vi "VI Execution Properties.vi"() -> ()   [LabVIEW 2023]
doc: "SubVI Inlining eliminates subVI calling overhead and enables additional optimizations, while maintaining source-code modularity. This example compares the run-time performance of an inline subVI against a normal subVI with debugging, a normal subVI without debugging, a subroutine subVI, and the primitive itself."
panel:
  out "Debugging Disabled":dbl
  out "Inlined":dbl
  out "Subroutine Priority":dbl
  out "Debugging Enabled":dbl
  out "Direct Function Call":dbl
  out "Data":dbl[](array[numeric])
  # "Overview: Demonstrates the performance effects of various VI Properties > Execution settings.\nInstructions:\n1. Close all open VIs except this one.\n2. Run the VI. It may take several seconds to complete. See the block diagram for more information on these benchmark values."
  # "Execution Times (ns)"
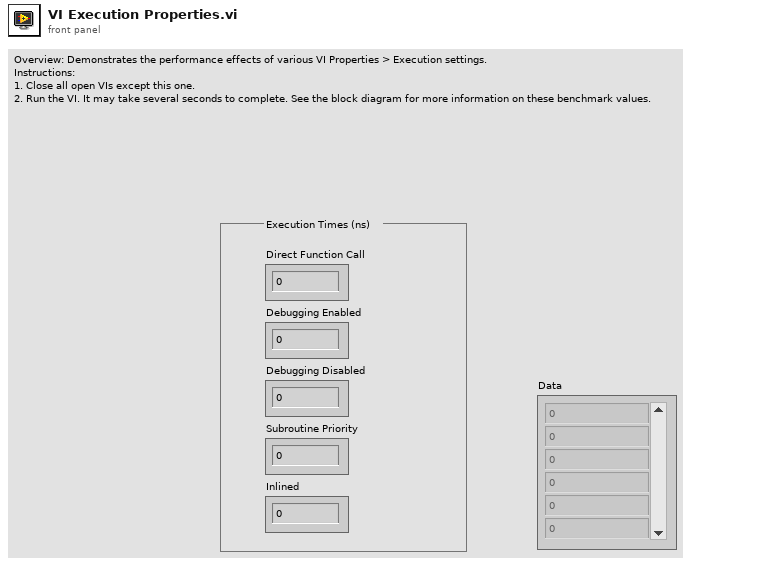
[diagram p1: front panel]
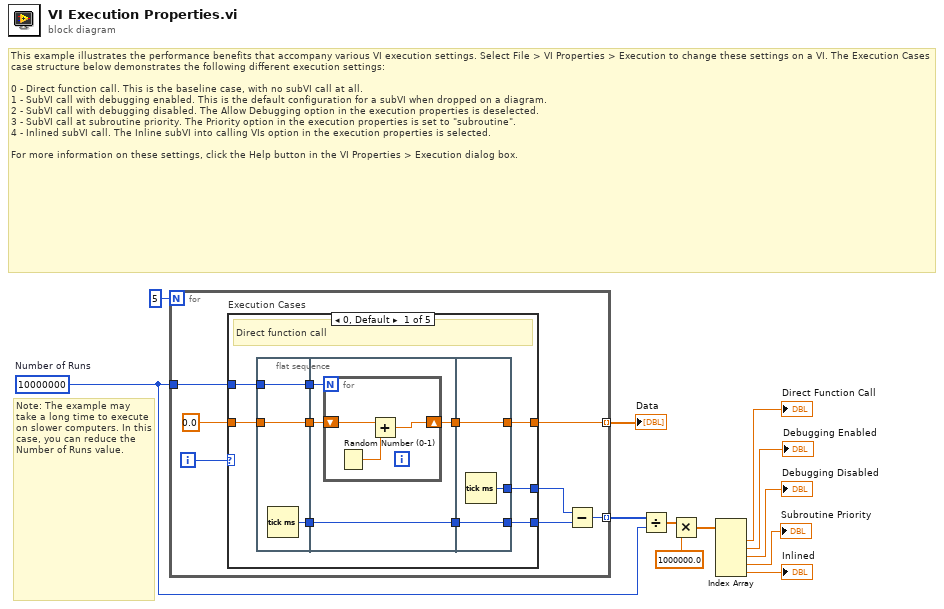
[diagram p0: block diagram]
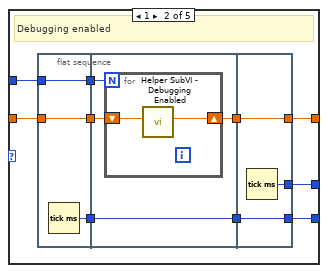
[diagram p2: hidden frame]
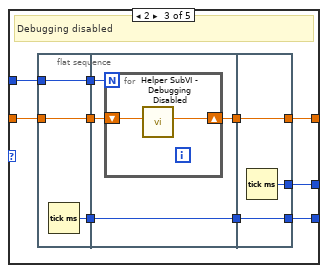
[diagram p3: hidden frame]
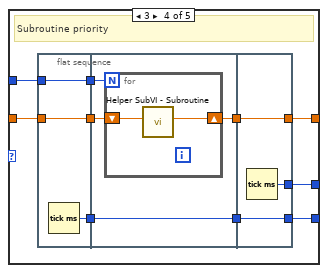
[diagram p4: hidden frame]
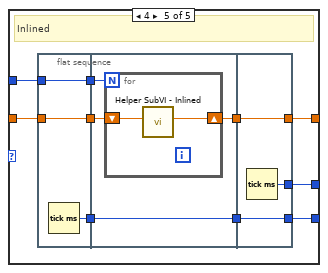
[diagram p5: hidden frame]
diagram:
  w10 = 10000000  # Number of Runs
  # "Note: The example may take a long time to execute on slower computers. In this case, you can reduce the Number of Runs value."
  # "This example illustrates the performance benefits that accompany various VI execution settings. Select File > VI Properties > Execution to change these settings on a VI. The Execution Cases case structure below demonstrates the following different execution settings:\n\n0 - Direct function call. This is the baseline case, with no subVI call at all.\n1 - SubVI call with debugging enabled. This is the default configuration for a subVI when dropped on a diagram.\n2 - SubVI call with debugging disabled. The Allow Debugging option in the execution properties is deselected.\n3 - SubVI call at subroutine priority. The Priority option in the execution properties is set to \"subroutine\".\n4 - Inlined subVI call. The Inline subVI into calling VIs option in the execution properties is selected.\n\nFor more information on these settings, click the Help button in the VI Properties > Execution dialog box."
  n1 = for {
    N: 5 -> [_]
    tunnel: [w17] -> w11 mode=indexing
    tunnel: w10 -> [w15]
    tunnel: [w16] -> w12 mode=indexing
    i -> [w13]
    n2 = case "Execution Cases" shown="0, Default" w13 {
      tunnel: [w24 w47 w69 w91 w113] -> w19
      tunnel: [w23 w46 w68 w90 w112] -> w18
      tunnel: [w22 w45 w67 w89 w111] -> w16
      tunnel: w15 -> [w21 w44 w66 w88 w110]
      tunnel: 0.0 -> [w20 w43 w65 w87 w109]
      frame 0, Default {
        # "Direct function call"
        n3 = flat-sequence {
          tunnel: [w32] -> w29
          tunnel: [w31] -> w28
          tunnel: w21 -> [w31]
          tunnel: [w30] -> w27
          tunnel: w20 -> [w30]
          tunnel: [w36] -> w26
          tunnel: w29 -> [w36]
          tunnel: w28 -> [w35]
          tunnel: w27 -> [w34]
          tunnel: [w33] -> w25
          tunnel: w26 -> [w42]
          tunnel: [w42] -> w23
          tunnel: [w41] -> w24
          tunnel: [w40] -> w22
          tunnel: w25 -> [w40]
          frame #0 {
            n4 = Tick Count (ms)() -> (millisecond timer value=w32:u32)
          }
          frame #1 {
            n5 = for {
              N: w35 -> [_]
              shift-right: [w38] -> w33
              shift-left: w34 -> [w39]
              n6 = Random Number (0-1)() -> (number: 0 to 1=w37:dbl)
              n7 = Add(x=w39, y=w37) -> (x+y=w38:dbl)
            }
          }
          frame #2 {
            n8 = Tick Count (ms)() -> (millisecond timer value=w41:u32)
          }
        }
      }
      frame 1 {
        # "Debugging enabled"
        n9 = flat-sequence {
          tunnel: [w55] -> w52
          tunnel: [w54] -> w51
          tunnel: w44 -> [w54]
          tunnel: [w53] -> w50
          tunnel: w43 -> [w53]
          tunnel: [w59] -> w49
          tunnel: w52 -> [w59]
          tunnel: w51 -> [w58]
          tunnel: w50 -> [w57]
          tunnel: [w56] -> w48
          tunnel: w49 -> [w64]
          tunnel: [w64] -> w46
          tunnel: [w63] -> w47
          tunnel: [w62] -> w45
          tunnel: w48 -> [w62]
          frame #0 {
            n10 = Tick Count (ms)() -> (millisecond timer value=w55:u32)
          }
          frame #1 {
            n11 = for {
              N: w58 -> [_]
              shift-right: [w60] -> w56
              shift-left: w57 -> [w61]
              n12 = call "Helper SubVI - Debugging Enabled.vi"("Numeric In"=w61) -> ("Numeric Out"=w60:dbl)  [unwired: 10 in]
            }
          }
          frame #2 {
            n13 = Tick Count (ms)() -> (millisecond timer value=w63:u32)
          }
        }
      }
      frame 2 {
        # "Debugging disabled"
        n14 = flat-sequence {
          tunnel: [w77] -> w74
          tunnel: [w76] -> w73
          tunnel: w66 -> [w76]
          tunnel: [w75] -> w72
          tunnel: w65 -> [w75]
          tunnel: [w81] -> w71
          tunnel: w74 -> [w81]
          tunnel: w73 -> [w80]
          tunnel: w72 -> [w79]
          tunnel: [w78] -> w70
          tunnel: w71 -> [w86]
          tunnel: [w86] -> w68
          tunnel: [w85] -> w69
          tunnel: [w84] -> w67
          tunnel: w70 -> [w84]
          frame #0 {
            n15 = Tick Count (ms)() -> (millisecond timer value=w77:u32)
          }
          frame #1 {
            n16 = for {
              N: w80 -> [_]
              shift-right: [w82] -> w78
              shift-left: w79 -> [w83]
              n17 = call "Helper SubVI - Debugging Disabled.vi"("Numeric In"=w83) -> ("Numeric Out"=w82:dbl)  [unwired: 10 in]
            }
          }
          frame #2 {
            n18 = Tick Count (ms)() -> (millisecond timer value=w85:u32)
          }
        }
      }
      frame 3 {
        # "Subroutine priority"
        n19 = flat-sequence {
          tunnel: [w99] -> w96
          tunnel: [w98] -> w95
          tunnel: w88 -> [w98]
          tunnel: [w97] -> w94
          tunnel: w87 -> [w97]
          tunnel: [w103] -> w93
          tunnel: w96 -> [w103]
          tunnel: w95 -> [w102]
          tunnel: w94 -> [w101]
          tunnel: [w100] -> w92
          tunnel: w93 -> [w108]
          tunnel: [w108] -> w90
          tunnel: [w107] -> w91
          tunnel: [w106] -> w89
          tunnel: w92 -> [w106]
          frame #0 {
            n20 = Tick Count (ms)() -> (millisecond timer value=w99:u32)
          }
          frame #1 {
            n21 = for {
              N: w102 -> [_]
              shift-right: [w104] -> w100
              shift-left: w101 -> [w105]
              n22 = call "Helper SubVI - Subroutine.vi"("Numeric In"=w105) -> ("Numeric Out"=w104:dbl)  [unwired: 10 in]
            }
          }
          frame #2 {
            n23 = Tick Count (ms)() -> (millisecond timer value=w107:u32)
          }
        }
      }
      frame 4 {
        # "Inlined"
        n24 = flat-sequence {
          tunnel: [w121] -> w118
          tunnel: [w120] -> w117
          tunnel: w110 -> [w120]
          tunnel: [w119] -> w116
          tunnel: w109 -> [w119]
          tunnel: [w125] -> w115
          tunnel: w118 -> [w125]
          tunnel: w117 -> [w124]
          tunnel: w116 -> [w123]
          tunnel: [w122] -> w114
          tunnel: w115 -> [w130]
          tunnel: [w130] -> w112
          tunnel: [w129] -> w113
          tunnel: [w128] -> w111
          tunnel: w114 -> [w128]
          frame #0 {
            n25 = Tick Count (ms)() -> (millisecond timer value=w121:u32)
          }
          frame #1 {
            n26 = for {
              N: w124 -> [_]
              shift-right: [w126] -> w122
              shift-left: w123 -> [w127]
              n27 = call "Helper SubVI - Inlined.vi"("Numeric In"=w127) -> ("Numeric Out"=w126:dbl)  [unwired: 10 in]
            }
          }
          frame #2 {
            n28 = Tick Count (ms)() -> (millisecond timer value=w129:u32)
          }
        }
      }
    }
    n29 = Subtract(x=w19, y=w18) -> (x-y=w17:u32)
  }
  "Data" <- w12
  n30 = Divide(x=w11, y=w10) -> (x/y=w9:dbl[])
  n31 = Multiply(x=w9, y=1000000.0) -> (x*y=w7:dbl[])
  n32 = Index Array(array=w7) -> (element #1=→"Direct Function Call":dbl, element #2=→"Debugging Enabled":dbl, element #3=→"Debugging Disabled":dbl, element #4=→"Subroutine Priority":dbl, element #5=→"Inlined":dbl)  [unwired: 5 in]
